vi "DrawTitle.vi"(8 "error in (no error)":errorcluster, 11 "Menu in":refnum<class "Menu.lvclass">) -> (0 "error out":errorcluster, 3 "Menu out":refnum<class "Menu.lvclass">)   [LabVIEW 2019, in "RT_Game.lvlib" / "Menu.lvclass"]
uses:
  Menu.lvclass
  C:/Users/FreshBob/Dropbox/VIs/myRIO_GameConsole/RT/RT_Game/Game/Game.lvclass
  Game/Coordinate.ctl
  Menu.lvclass/Menu.ctl
  Game/Game.lvclass
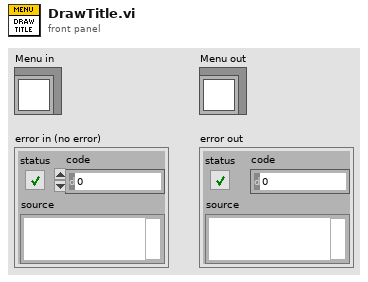
[diagram p1: front panel]
types:
  T1 = typedef "RT_Game.lvlib/Game.lvclass/Coordinate.ctl" = cluster{"x":dbl, "y":dbl}
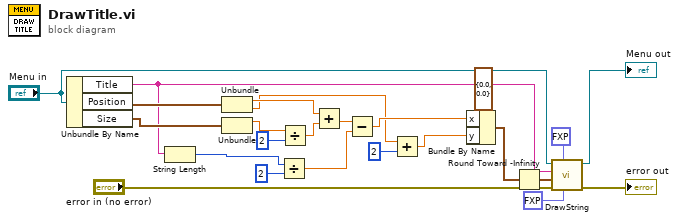
[diagram p0: block diagram]
diagram:
  n1 = Unbundle By Name("Menu in") -> ("Title"=w13:string, "Position"=w18:T1, "Size"=w17:T1)
  n2 = String Length(string=w13) -> (length=w9:i32)
  n3 = Unbundle(w18) -> ("x"=w15:dbl, "y"=w6:dbl)
  n4 = Unbundle(w17) -> ("x"=w16:dbl)  [unwired: 1 out]
  n5 = Divide(x=w9, y=i16 2) -> (x/y=w8:dbl)
  n6 = Divide(x=w16, y=i16 2) -> (x/y=w14:dbl)
  n7 = Add(x=w15, y=w14) -> (x+y=w12:dbl)
  n8 = Subtract(x=w12, y=w8) -> (x-y=w7:dbl)
  n9 = Add(x=w6, y=i16 2) -> (x+y=w5:dbl)
  n10 = Bundle By Name(cluster=T1 {"x"=0.0, "y"=0.0} ("y"), "x"=w7, "y"=w5) -> (w20:T1)
  n11 = Round Toward -Infinity(1:w20) -> (0:w3:T1)
  n12 = call "DrawString.vi"("ColorToReplace (7=white)"=fxp<+,3,3> 5.0, "Color (7=white)"=fxp<+,3,3> 1.0, "error in (no error)"="error in (no error)", "Coordinate"=w3, "String"=w13, "RT_Game.lvlib:Game.lvclass"="Menu in") -> ("error out"=→"error out":errorcluster, "RT_Game.lvlib:Game.lvclass 2"=→"Menu out":refnum<class "Menu.lvclass">)  [unwired: 4 in]
